vi "test.vi"() -> ()   [LabVIEW 2016]
uses:
  Electrometer.lvclass
panel:
  out "Waveform Chart":dbl(graph)
  in  "stop":bool
  out "Volt":dbl
  out "error out":errorcluster
  in  "VISA":refnum<visa-resource-name>
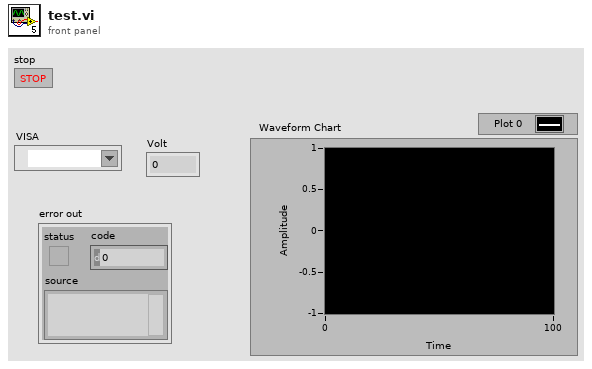
[diagram p1: front panel]
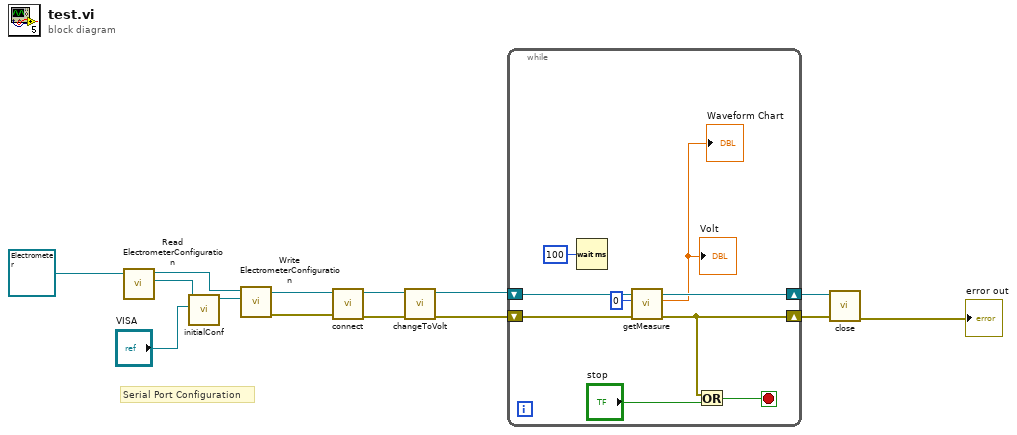
[diagram p0: block diagram]
diagram:
  # "Serial Port Configuration"
  n1 = call-dynamic "Read ElectrometerConfiguration.vi"("Electrometer in"=refnum<class "Electrometer.lvclass"> refnum ("Electrometer.lvclass")) -> ("ElectrometerConfiguration.lvclass"=w13:refnum<class "ElectrometerConfiguration.lvclass">, "Electrometer out"=w10:refnum<class "Electrometer.lvclass">)  [unwired: 8 in, 1 out]
  n2 = call "initialConf.vi"("VISA"="VISA", "ElectrometerConfiguration.lvclass"=w13) -> ("ElectrometerConfiguration"=w11:refnum<class "ElectrometerConfiguration.lvclass">)  [unwired: 9 in]
  n3 = call-dynamic "Write ElectrometerConfiguration.vi"("ElectrometerConfiguration.lvclass"=w11, "Electrometer in"=w10) -> ("error out"=w6:errorcluster, "Electrometer out"=w5:refnum<class "Electrometer.lvclass">)  [unwired: 8 in]
  n4 = call "connect.vi"("error in (no error)"=w6, "Electrometer in"=w5) -> ("error out"=w4:errorcluster, "Electrometer out"=w2:refnum<class "Electrometer.lvclass">)  [unwired: 7 in, 1 out]
  n5 = call-dynamic "changeToVolt.vi"("error in (no error)"=w4, "Electrometer in"=w2) -> ("error out"=w3:errorcluster, "Electrometer out"=w1:refnum<class "Electrometer.lvclass">)  [unwired: 8 in]
  n6 = while {
    shift-right: [w20] -> w7
    shift-left: w1 -> [w23]
    shift-right: [w15] -> w9
    shift-left: w3 -> [w22]
    stop <- w17 stop-if-true
    n7 = Wait (ms)(milliseconds to wait=u32 100) -> ()  [unwired: 1 out]
    n8 = call-dynamic "getMeasure.vi"("error in (no error)"=w22, "Reading Option (0: Latest)"=0, "Electrometer in"=w23) -> ("error out"=w15:errorcluster, "Measure"=→"Volt" →"Waveform Chart":dbl, "Electrometer out"=w20:refnum<class "Electrometer.lvclass">)  [unwired: 6 in]
    n9 = Or(x=w15, y="stop") -> (x .or. y?=w17:bool)
  }
  n10 = call "close.vi"("error in (no error)"=w9, "Electrometer in"=w7) -> ("error out"=→"error out":errorcluster)  [unwired: 8 in, 1 out]
